vi "initial-连接数据库-加载企业与用户列表.vi"(10 "数据库连接信息":T1={"登录名"="sa", "密码"="xjr.1993215", "初始数据库"="master"}, 11 "个人剂量仪-云服务器.i":refnum<class "个人剂量仪-云服务器.lvclass">) -> (2 "成功？":bool, 3 "个人剂量仪-云服务器.o":refnum<class "个人剂量仪-云服务器.lvclass">)   [LabVIEW 2013, in "个人剂量仪-云服务器.lvclass"]
doc: "此VI连接本地服务器，并加载所有‘企业文件夹’下的企业信息，与对应的企业数据库中的所有用户列表。"
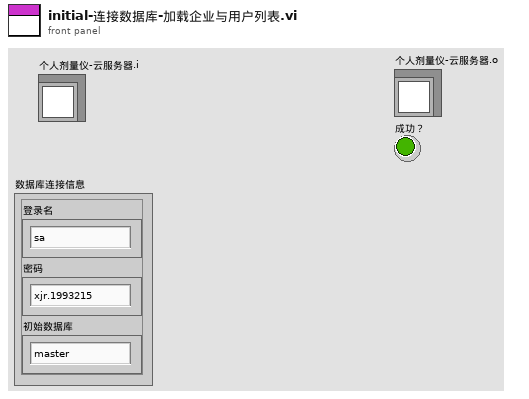
[diagram p1: front panel]
types:
  T1 = cluster{"登录名":string, "密码":string, "初始数据库":string}
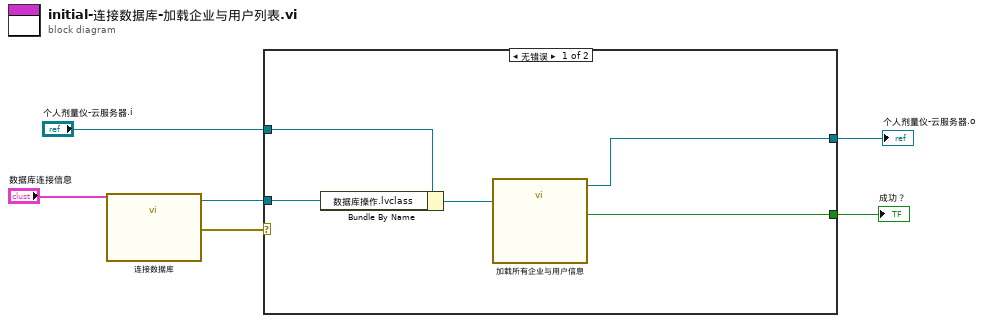
[diagram p0: block diagram]
diagram:
  n1 = call "连接数据库.vi"("数据库连接信息"="数据库连接信息") -> ("error out"=w3:errorcluster, "obj-数据库操作 o"=w2:refnum<class "数据库操作.lvclass">)  [unwired: 9 in]
  n2 = case shown="无错误" w3 {
    tunnel: "个人剂量仪-云服务器.i" -> [w11 w12]
    tunnel: [w8 w12] -> w4
    tunnel: w2 -> [w10 _]
    tunnel: [w7 _] -> w1
    frame No Error {
      n3 = Bundle By Name(cluster=w11, "数据库操作.lvclass"=w10) -> (w9:refnum<class "个人剂量仪-云服务器.lvclass">)
      n4 = call "加载所有企业与用户信息.vi"("个人剂量仪-云服务器.i"=w9) -> ("获取成功？"=w7:bool, "个人剂量仪-云服务器.o"=w8:refnum<class "个人剂量仪-云服务器.lvclass">)  [unwired: 9 in]
    }
    frame Error {
    }
  }
  "个人剂量仪-云服务器.o" <- w4
  "成功？" <- w1
